vi "AppClose.vi"(8 "error in (no error)":errorcluster) -> ()   [LabVIEW 2016]
uses:
  Tools/Translator/Translator.Control.Fglb.Action.vi
  Tools/Translator/Translator.Message.ctl
  Tools/EventLog/EventLog.New(single).vi
  Global/ApplicationGlobal.vi
  Tools/EventLog/EventLog.Buffer.vi
  Tools/EventLog/EventLog.File.ReadWrite.vi
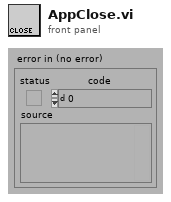
[diagram p1: front panel]
types:
  T1 = typedef "Translator.Control.Fglb.Action.vi" = enum16{"init", "set", "get", "clear"}
  T2 = typedef "Translator.Message.ctl" = enum16{"-", "Event confirmed", "Log out", "Log in", "Shutdown", "Cancel", "Start", "Continue", "Stop", "On", "Off", "OK", "NOK", "NOK %s", "This", "Prev", "Home", "Work", "In progress...", "Missing", "Empty", "Hardware failure", "Initial", "Error %d >> %s", "Error %d >> %s >> %s", "Starting %s", "Quitting %s", "Configured", "Initializing", "Quitting", "Loading", "Running %s", "Stopped", "Summary", "Do you want to continue?", "Do you want to exit?", "Log out?", "System", "All", "IDLE", "Translating...%s", "Not found", "Alarm %s", "Run", "Skip", "Abort", "Repeat", "Please wait...", "Database disconnected", "Login to database successful", "Login to database failed: %d; %s", "Get process step data for %s", "Changeover off", "Changeover into %s", "Product %s | %s found in cache with status %d at previous station", "Product %s | %s found in database with status %d at previous station", "Product %s | %s not found in cache at previous station", "Product %s | %s not found in database at previous station", "Product %s | %s found in cache with status %d at this station (%d repetion)", "Product %s | %s found in database with status %d at this station (%d repetition)", "Product %s | %s not found in cache at this station", "Product %s | %s not found in database at this station", "Product %s | %s found in cache for component %s | %s", "Product %s | %s found in database for component %s | %s", "Product not found in cache for component %s | %s", "Product not found in database for component %s | %s", "Product %s | %s connected with component %s | %s (cache)", "Product %s | %s connected with component %s | %s (database)", "New data for %s | %s (cache)", "New data for %s | %s (database)", "File %s moved (cache)", "File %s deleted (cache)", "Msg %d >> %s", "PLC LifeBit Failure", "Reconnecting DB", "Reconnecting PLC", "Free disk space is below 1GB - contact technician", "Unable to check product status", "Product %s SN %s checked in DB", "Unable To check status from station %s"}
  T3 = typedef "Windows.ExitAction.ctl" = enum16{"Log off from PC", "Shut Down PC", "Reboot PC", "Close Program"}
  T4 = enum32{"invalid app kind", "Development System", "Run Time System", "Student Edition", "Embedded LabVIEW", "Evaluation", "Custom"}
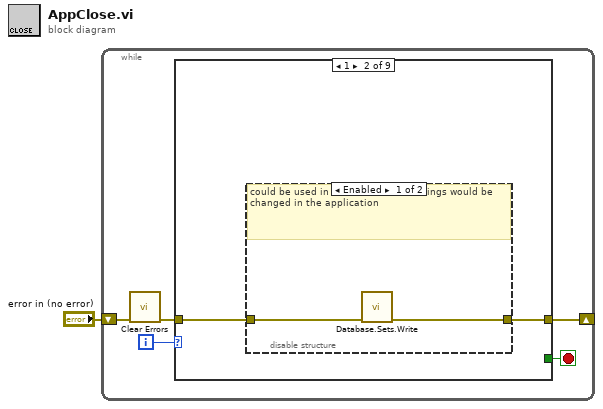
[diagram p0: block diagram]
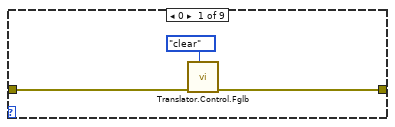
[diagram p2: hidden frame]
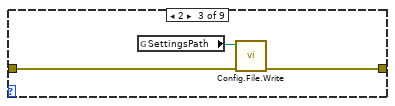
[diagram p4: hidden frame]
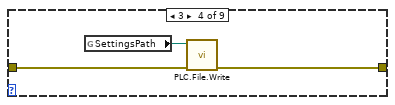
[diagram p5: hidden frame]
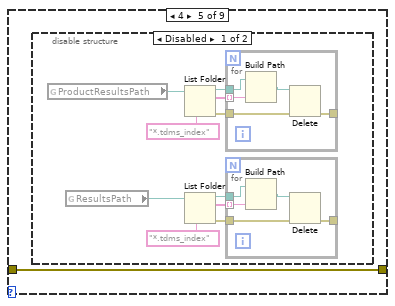
[diagram p6: hidden frame]
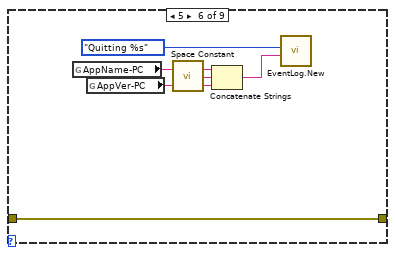
[diagram p8: hidden frame]
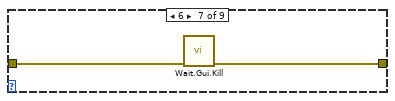
[diagram p9: hidden frame]
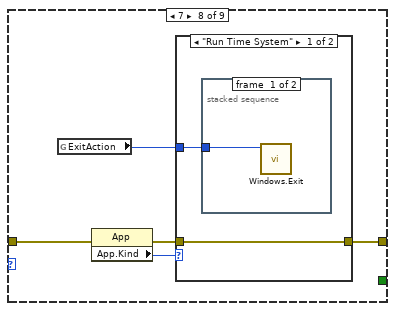
[diagram p10: hidden frame]
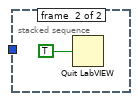
[diagram p11: hidden frame]
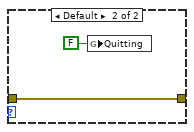
[diagram p12: hidden frame]
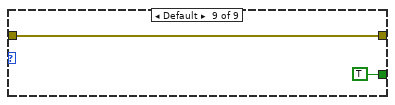
[diagram p13: hidden frame]
diagram:
  n1 = while {
    shift-right: [w2] -> _
    shift-left: "error in (no error)" -> [w4]
    i -> [w6]
    stop <- w5 stop-if-true
    n2 = call <vilib>:"Clear Errors.vi"("error in (no error)"=w4) -> ("error out"=w3:errorcluster)  [unwired: 5 in, 1 out]
    n3 = case shown="1" w6 {
      tunnel: [_ _ _ _ _ _ _ _ TRUE] -> w5
      tunnel: w3 -> [w8 w11 w16 w19 w21 w47 w49 w51 w61]
      tunnel: [w7 w10 w17 w18 w21 w47 w48 w50 w61] -> w2
      frame 0 {
        n4 = call "Translator.Control.Fglb.vi"("Action"=Translator.Control.Fglb.Action.vi."clear", "error in (no error)"=w8) -> ("error out"=w7:errorcluster)  [unwired: 8 in, 1 out]
      }
      frame 1 {
        n5 = disable-structure shown="Enabled" {
          disable-tunnel: w11 -> [w13 w14]
          disable-tunnel: [w12 w14] -> w10
          frame Enabled {
            # "could be used in the future if DB settings would be changed in the application"
            n6 = call "Database.Sets.Write.vi"("error in"=w13) -> ("error out"=w12:errorcluster)  [unwired: 10 in]
          }
          frame Disabled {
          }
        }
      }
      frame 2 {
        n7 = global read "ApplicationGlobal.vi" "SettingsPath"() -> (w15:path)
        n8 = call "Config.File.Write.vi"("error in"=w16, "path"=w15) -> ("error out"=w17:errorcluster)  [unwired: 9 in]
      }
      frame 3 {
        n9 = global read "ApplicationGlobal.vi" "SettingsPath"() -> (w20:path)
        n10 = call "PLC.File.Write.vi"("error in"=w19, "path"=w20) -> ("error out"=w18:errorcluster)  [unwired: 9 in]
      }
      frame 4 {
        n11 = disable-structure shown="Disabled" {
          frame Disabled {
            n12 = global read "ApplicationGlobal.vi" "ProductResultsPath"() -> (w31:path)
            n13 = global read "ApplicationGlobal.vi" "ResultsPath"() -> (w22:path)
            n14 = List Folder(path=w31, pattern="*.tdms_index") -> (path out=w27:path, filenames=w28:string[], error out=w29:errorcluster)  [unwired: 2 in, 1 out]
            n15 = List Folder(path=w22, pattern="*.tdms_index") -> (path out=w26:path, filenames=w25:string[], error out=w24:errorcluster)  [unwired: 2 in, 1 out]
            n16 = for {
              tunnel: w29 -> [w38]
              tunnel: w28 -> [w41] mode=indexing
              tunnel: w27 -> [w40]
              tunnel: [w37] -> _
              n17 = Build Path(base path=w40, name or relative path=w41) -> (appended path=w39:path)
              n18 = Delete(path (use dialog)=w39, error in=w38) -> (error out=w37:errorcluster)  [unwired: 3 in, 2 out]
            }
            n19 = for {
              tunnel: w24 -> [w33]
              tunnel: w25 -> [w36] mode=indexing
              tunnel: w26 -> [w35]
              tunnel: [w32] -> _
              n20 = Build Path(base path=w35, name or relative path=w36) -> (appended path=w34:path)
              n21 = Delete(path (use dialog)=w34, error in=w33) -> (error out=w32:errorcluster)  [unwired: 3 in, 2 out]
            }
          }
          frame Enabled {
          }
        }
      }
      frame 5 {
        n22 = global read "ApplicationGlobal.vi" "AppName-PC"() -> (w45:string)
        n23 = global read "ApplicationGlobal.vi" "AppVer-PC"() -> (w44:string)
        n24 = call <vilib>:"Space Constant.vi"() -> ("String"=w43:string)
        n25 = Concatenate Strings(w45, w43, w44) -> (w42:string)
        n26 = call-poly "EventLog.New.vi"("Arg"=w42, "Message (-)"=Translator.Message."Quitting %s") -> ()  [unwired: 8 in, 2 out]
      }
      frame 6 {
        n27 = call "Wait.Gui.Kill.vi"("error in (no error)"=w49) -> ("error out"=w48:errorcluster)  [unwired: 10 in]
      }
      frame 7 {
        n28 = global read "ApplicationGlobal.vi" "ExitAction"() -> (w52:T3)
        n29 = property class="App"(error in=w51) -> (error out=w53:errorcluster, "App.Kind"=w54:T4)  [unwired: 1 in, 1 out]
        n30 = case shown="\"Run Time System\"" w54 {
          tunnel: w53 -> [w55 w60]
          tunnel: w52 -> [w56 _]
          tunnel: [w55 w60] -> w50
          frame "Run Time System" {
            n31 = stacked-sequence {
              tunnel: w56 -> [w57 _]
              frame #0 {
                n32 = call "Windows.Exit.vi"("Exit Action"=w57) -> ()  [unwired: 6 in, 1 out]
              }
              frame #1 {
                n33 = Quit LabVIEW(quit? (T)=TRUE) -> ()
              }
            }
          }
          frame Default {
            n34 = global write "ApplicationGlobal.vi" "Quitting"(FALSE ("Quitting")) -> ()
          }
        }
      }
      frame Default {
      }
    }
  }
